vi "Test Basic Operations Sin Cos.vi"() -> ()   [LabVIEW 2014, in "Complex Numbers.lvlib"]
uses:
  Complex Numbers.lvlib
  <vilib>/Aledyne-TSXperts/Arduino Compatible Compiler for LabVIEW/Arduino Compatible Compiler for LabVIEW.lvlib
panel:
  out "error out":errorcluster
  in  "error in (no error)":errorcluster
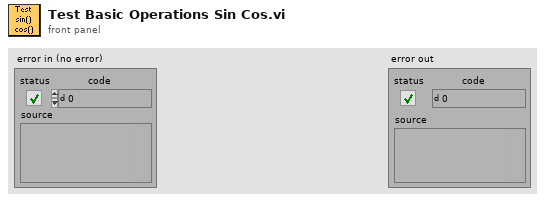
[diagram p1: front panel]
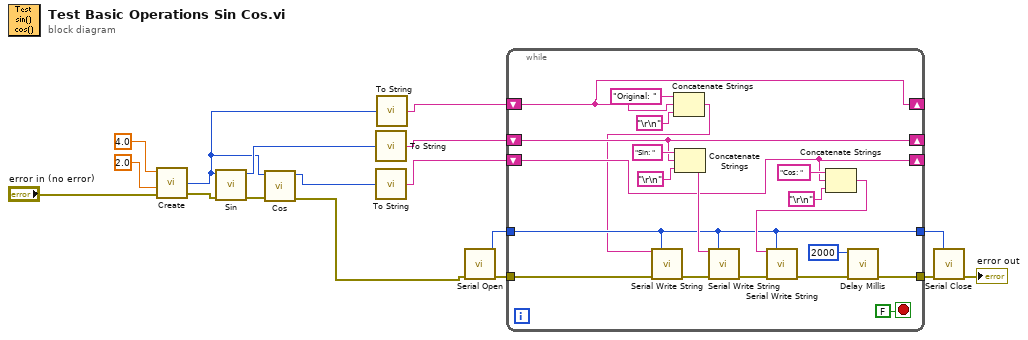
[diagram p0: block diagram]
diagram:
  n1 = call "Create.vi"("Error In"="error in (no error)", "Imag"=2.0, "Real"=4.0) -> ("Error Out"=w7:errorcluster, "Complex"=w2:u32)  [unwired: 2 in]
  n2 = call "Sin.vi"("Error In"=w7, "A"=w2) -> ("Error Out"=w6:errorcluster, "sin(A)"=w3:u32)  [unwired: 8 in]
  n3 = call "Cos.vi"("Error In"=w6, "A"=w2) -> ("Error Out"=w5:errorcluster, "sin(A)"=w4:u32)  [unwired: 8 in]
  n4 = call "To String.vi"("Complex number"=w3) -> ("String complex num."=w8:string)
  n5 = call "To String.vi"("Complex number"=w4) -> ("String complex num."=w9:string)
  n6 = call "To String.vi"("Complex number"=w2) -> ("String complex num."=w1:string)
  n7 = call <vilib>:"Serial Open.vi"("error in (no error)"=w5) -> ("Instance"=w15:u8, "error out"=w17:errorcluster)  [unwired: 13 in]
  n8 = while {
    tunnel: w17 -> [w23]
    tunnel: [w35] -> w16
    tunnel: w15 -> [w22]
    tunnel: [w22] -> w14
    shift-right: [w27] -> _
    shift-left: w8 -> [w27]
    shift-right: [w25] -> _
    shift-left: w9 -> [w25]
    shift-right: [w19] -> _
    shift-left: w1 -> [w19]
    stop <- FALSE stop-if-true
    n9 = Concatenate Strings("Original: " ("string"), w19, "\r\n") -> (w18:string)
    n10 = call <vilib>:"Serial Write String.vi"("String"=w18, "Instance"=w22, "error in (no error)"=w23) -> ("error out"=w24:errorcluster)  [unwired: 12 in]
    n11 = Concatenate Strings("Sin: " ("string"), w27, "\r\n") -> (w30:string)
    n12 = call <vilib>:"Serial Write String.vi"("String"=w30, "Instance"=w22, "error in (no error)"=w24) -> ("error out"=w33:errorcluster)  [unwired: 12 in]
    n13 = Concatenate Strings("Cos: " ("string"), w25, "\r\n") -> (w29:string)
    n14 = call <vilib>:"Serial Write String.vi"("String"=w29, "Instance"=w22, "error in (no error)"=w33) -> ("error out"=w36:errorcluster)  [unwired: 12 in]
    n15 = call <vilib>:"Delay Millis.vi"("error in (no error)"=w36, "delay"=u32 2000) -> ("error out"=w35:errorcluster)  [unwired: 9 in]
  }
  n16 = call <vilib>:"Serial Close.vi"("Instance"=w14, "error in (no error)"=w16) -> ("error out"=→"error out":errorcluster)  [unwired: 13 in]
